vi "Decode (Single Param).vi"(10 "parameter configuration":T1, 11 "Word in":u16) -> (2 "Parameter Value out":dbl, 3 "Word out":u16)   [LabVIEW 2020]
uses:
  _typedefs/parameter_config_type.ctl
  _typedefs/parameter_config_type_type.ctl
  _typedefs/parameter_config_encoding_type.ctl
  datatypes/dt_encodeDecode.lvlib
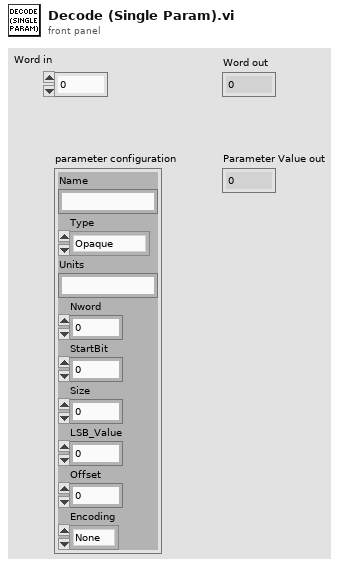
[diagram p1: front panel]
types:
  T1 = typedef "parameter_config_type.ctl" = cluster{"Name":string, "Type":T2, "Units":string, "Nword":i32, "StartBit":i32, "Size":i32, "LSB_Value":dbl, "Offset":i32, "Encoding":T3}
  T2 = typedef "parameter_config_type_type.ctl" = enum16{"Opaque", "Enum", "Float", "Integer", "Bcd", "Bool"}
  T3 = typedef "parameter_config_encoding_type.ctl" = enum16{"None", "2-complement", "Unsigned"}
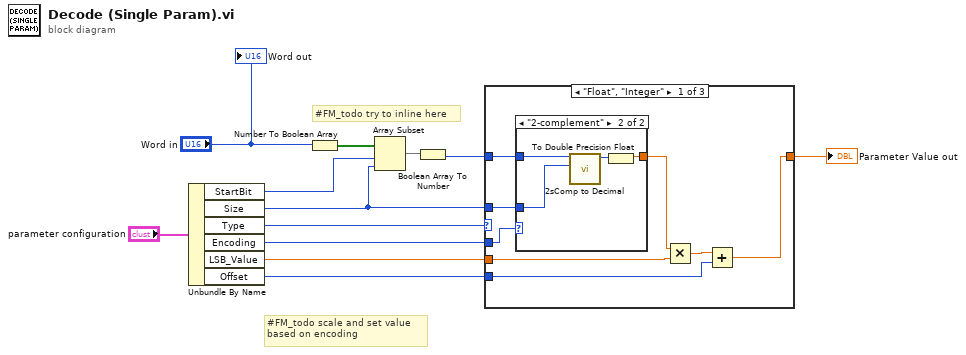
[diagram p0: block diagram]
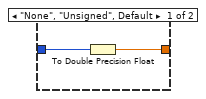
[diagram p2: hidden frame]
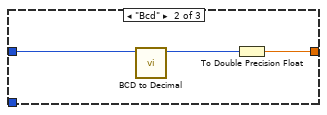
[diagram p3: hidden frame]
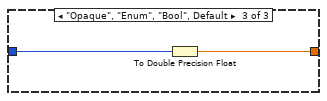
[diagram p4: hidden frame]
diagram:
  # "#FM_todo scale and set value \nbased on encoding"
  # "#FM_todo try to inline here"
  n1 = Unbundle By Name("parameter configuration") -> ("StartBit"=w10:i32, "Size"=w1:i32, "Type"=w7:T2, "Encoding"=w2:T3, "LSB_Value"=w3:dbl, "Offset"=w4:i32)
  n2 = Number To Boolean Array(number="Word in") -> (Boolean array=w9:bool[])
  n3 = Array Subset(array=w9, index=w10, length=w1) -> (w8:bool[])
  n4 = Boolean Array To Number(Boolean array=w8) -> (number=w6:u16)
  n5 = case shown="\"Float\", \"Integer\"" w7 {
    tunnel: w6 -> [w14 w29 w31]
    tunnel: [w19 w27 w30] -> w5
    tunnel: w4 -> [w18 _ _]
    tunnel: w3 -> [w17 _ _]
    tunnel: w2 -> [w16 _ _]
    tunnel: w1 -> [w13 _ _]
    frame "Float", "Integer" {
      n6 = case shown="\"2-complement\"" w16 {
        tunnel: [w21 w23] -> w15
        tunnel: w14 -> [w22 w26]
        tunnel: w13 -> [_ w25]
        frame "None", "Unsigned", Default {
          n7 = To Double Precision Float(number=w22) -> (double precision float=w21:dbl)
        }
        frame "2-complement" {
          n8 = call "2sComp to Decimal.vi"("size in bit"=w25, "word in"=w26) -> ("decimal out"=w24:i16)  [unwired: 9 in]
          n9 = To Double Precision Float(number=w24) -> (double precision float=w23:dbl)
        }
      }
      n10 = Multiply(x=w15, y=w17) -> (x*y=w20:dbl)
      n11 = Add(x=w20, y=w18) -> (x+y=w19:dbl)
    }
    frame "Bcd" {
      n12 = call "BCD to Decimal.vi"("word raw data - bcd"=w29) -> ("decimal data out"=w28:u32)  [unwired: 10 in]
      n13 = To Double Precision Float(number=w28) -> (double precision float=w27:dbl)
    }
    frame "Opaque", "Enum", "Bool", Default {
      n14 = To Double Precision Float(number=w31) -> (double precision float=w30:dbl)
    }
  }
  "Parameter Value out" <- w5
  "Word out" <- "Word in"
